vi "practica2.vi"() -> ()   [LabVIEW 2013]
panel:
  out "Waveform Chart":dbl(graph)
  in  "Encender":bool
  in  "Practica brazo robotico":string
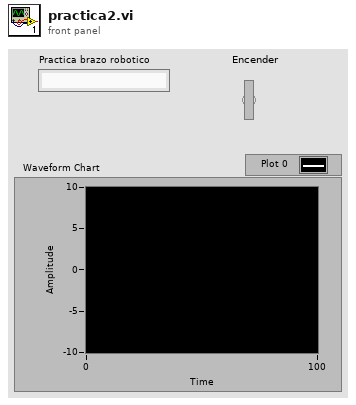
[diagram p1: front panel]
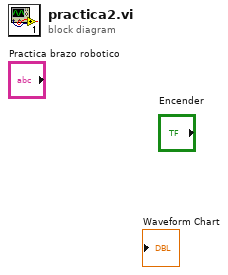
[diagram p0: block diagram]
diagram:
